vi "AutoHoldCan.vi"() -> (0 "Done?":bool)   [LabVIEW 2014]
uses:
  Robot Global Data.vi
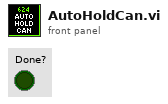
[diagram p1: front panel]
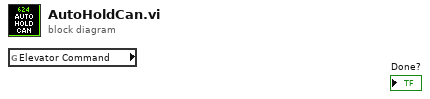
[diagram p0: block diagram]
diagram:
  n1 = global read "Robot Global Data.vi" "Elevator Command"() -> ()  [unwired: 1 out]
